vi "Set Initialization Data - TCPServer.vi"(8 "error in":errorcluster, 11 "Debug Server in":refnum<class "Debug Server.lvclass">) -> (0 "error out":errorcluster, 3 "Debug Server out":refnum<class "Debug Server.lvclass">)   [LabVIEW 2017, in "Debug Server.lvclass"]
doc: "Sets the initialization data of a statically linked subWorker."
uses:
  Debug Server.lvclass
  Debug Server TCP Server and Client/Workers/DS TCP Server/Initialization Data.ctl
  Debug Server TCP Server and Client/Workers/DS TCP Server/Response Cases.ctl
  <vilib>/addons/_Workers/Library/Case Label.ctl
  Debug Server.lvclass/Debug Server.ctl
  Debug Server TCP Server and Client/Workers/DS TCP Server/DS TCP Server.lvclass
  C:/Program Files (x86)/National Instruments/LabVIEW 2017/vi.lib/addons/_Workers/Library/Classes/Worker/Worker.lvclass
  <vilib>/addons/_Workers/Library/Workers.lvlib
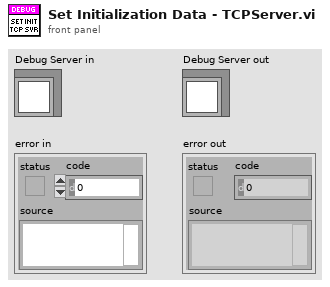
[diagram p1: front panel]
types:
  T1 = typedef "DS TCP Server.lvlib/DS TCP Server.lvclass/Initialization Data.ctl" = cluster{"Response Cases":T2}
  T2 = typedef "DS TCP Server.lvlib/DS TCP Server.lvclass/Response Cases.ctl" = cluster{"Server Port Open":T3, "Connection Notify":T3, "Incompatible DC Connection":T3}
  T3 = typedef "Workers.lvlib/Case Label.ctl" = string
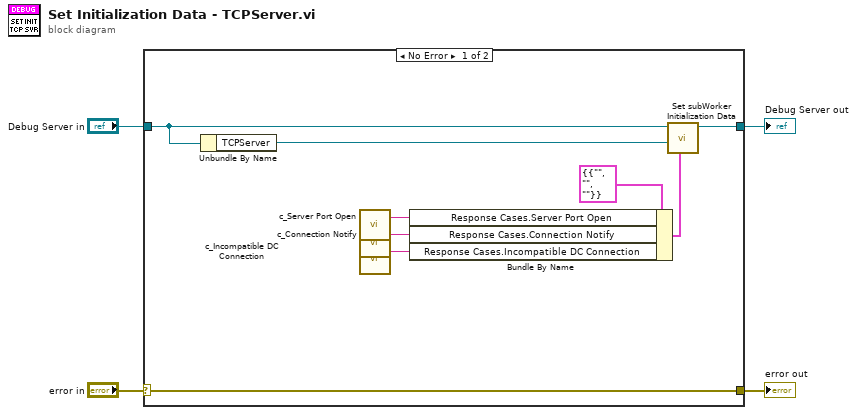
[diagram p0: block diagram]
diagram:
  n1 = case shown="No Error" "error in" {
    selector: "error in" -> [w13 w15]
    tunnel: [w13 w15] -> w3
    tunnel: [w11 w14] -> w2
    tunnel: "Debug Server in" -> [w10 w14]
    frame No Error {
      n2 = Unbundle By Name(w10) -> ("TCPServer"=w12:refnum<class "DS TCP Server.lvclass">)
      n3 = call "c_Server Port Open.vi"() -> ("Case Label"=w7:T3)  [unwired: 1 in]
      n4 = call "c_Connection Notify.vi"() -> ("Case Label"=w6:T3)  [unwired: 1 in]
      n5 = call "c_Incompatible DC Connection.vi"() -> ("Case Label"=w5:T3)  [unwired: 1 in]
      n6 = Bundle By Name(cluster=T1 {"Response Cases"={"Server Port Open"="", "Connection Notify"="", "Incompatible DC Connection"=""}} ("Initialization Data"), "Response Cases.Server Port Open"=w7, "Response Cases.Connection Notify"=w6, "Response Cases.Incompatible DC Connection"=w5) -> (w8:T1)
      n7 = call-dynamic "Set subWorker Initialization Data.vi"("Initialization Data"=w8, "subWorker"=w12, "Worker"=w10) -> ("Worker out"=w11:refnum<class "Debug Server.lvclass">)  [unwired: 8 in]
    }
    frame Error {
    }
  }
  "error out" <- w3
  "Debug Server out" <- w2
